vi "Load Layout By Name.vi"(8 "error in (no error)":errorcluster, 10 "key":string, 11 "Cluster":T6) -> (0 "error out":errorcluster)   [LabVIEW 2020, in "MDI ViewManager.lvlib"]
uses:
  MDI ViewManager.lvlib
  Typedef/Layout.ctl
  <vilib>/Utility/miscctls.llb/LVPointTypeDef.ctl
  <vilib>/Utility/miscctls.llb/LVBoundsTypeDef.ctl
  <vilib>/Utility/miscctls.llb/LVPositionTypeDef.ctl
  Typedef/Update View.ctl
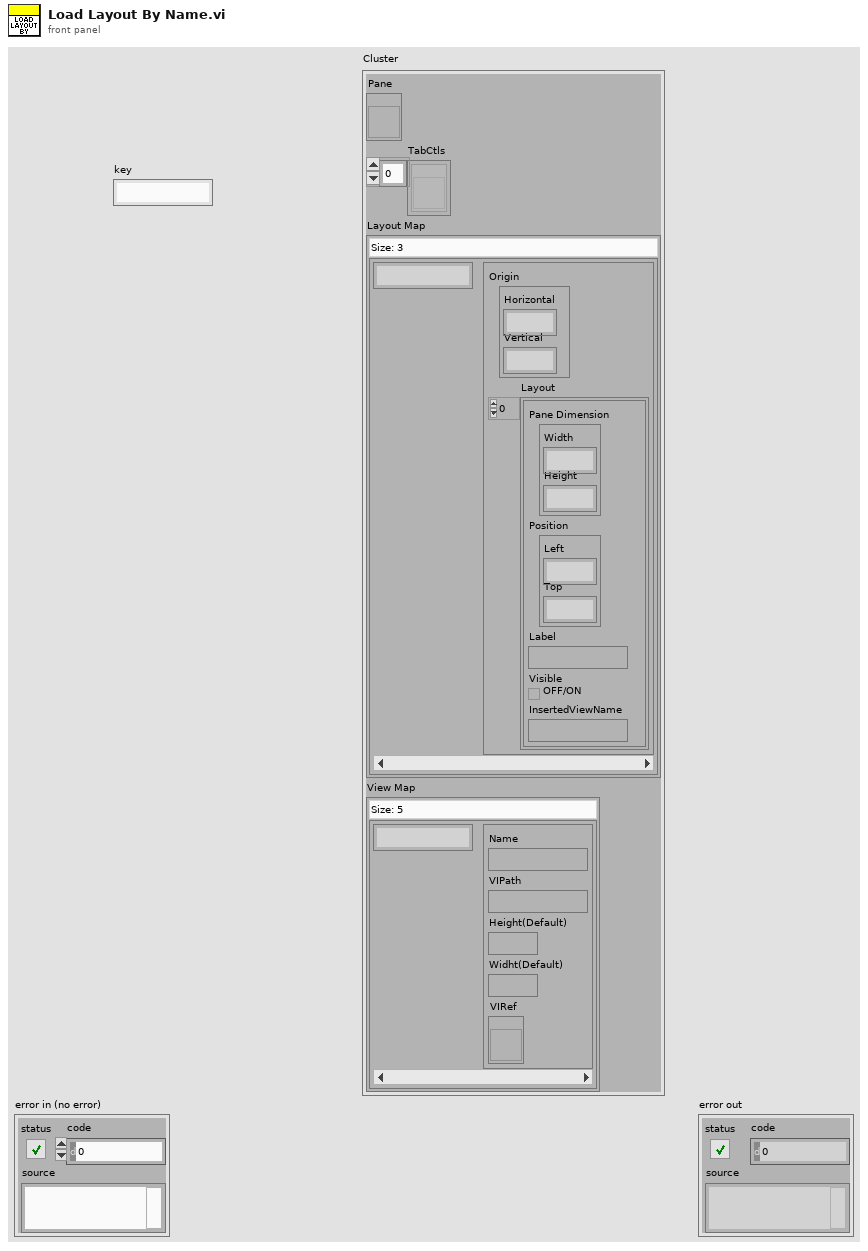
[diagram p1: front panel]
types:
  T1 = typedef "MDI ViewManager.lvlib/Layout.ctl" = cluster{"Origin":T2, "Layout":cluster{"Pane Dimension":T3, "Position":T4, "Label":string, "Visible":bool, "InsertedViewName":string}[]}
  T2 = typedef "LVPointTypeDef.ctl" = cluster{"Horizontal":i16, "Vertical":i16}
  T3 = typedef "LVBoundsTypeDef.ctl" = cluster{"Width":u32, "Height":u32}
  T4 = typedef "LVPositionTypeDef.ctl" = cluster{"Left":i32, "Top":i32}
  T5 = typedef "MDI ViewManager.lvlib/Update View.ctl" = cluster{"Name":string, "VIPath":path, "Height(Default)":u32, "Widht(Default)":u32, "VIRef":refnum<vi>}
  T6 = cluster{"Pane":refnum<vi>, "TabCtls":refnum<vi>[], "Layout Map":map{string, T1}, "View Map":map{string, T5}}
  T7 = cluster{"Pane Dimension":T3, "Position":T4, "Label":string, "Visible":bool, "InsertedViewName":string}[]
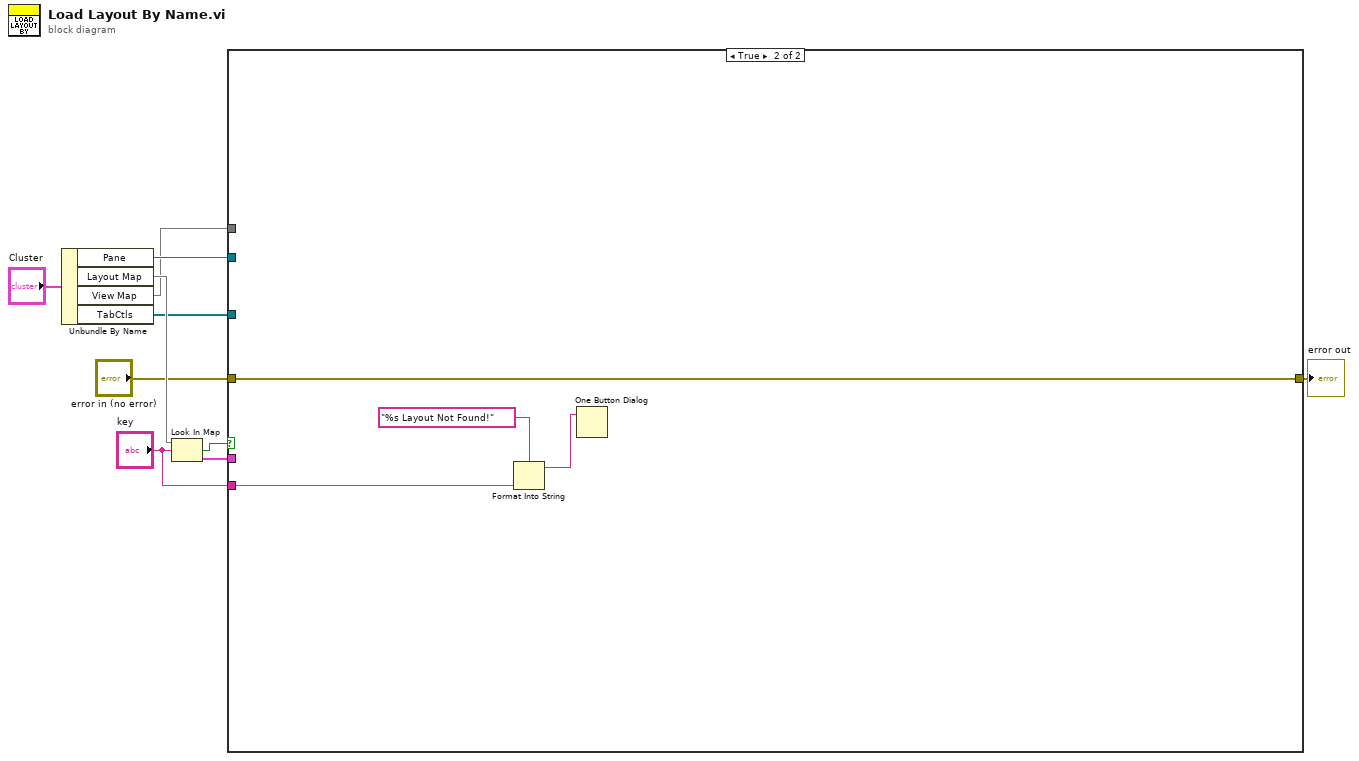
[diagram p0: block diagram]
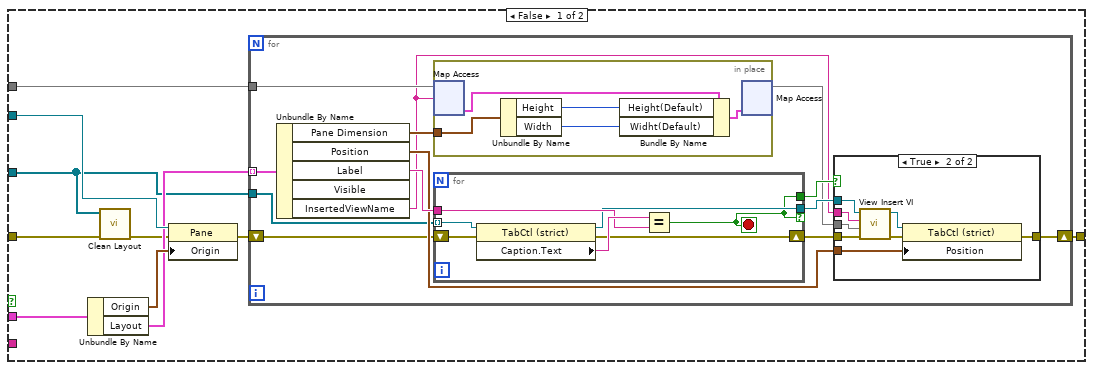
[diagram p2: hidden frame]
diagram:
  n1 = Unbundle By Name("Cluster") -> ("Pane"=w9:refnum<vi>, "Layout Map"=w8:map{string, T1}, "View Map"=w6:map{string, T5}, "TabCtls"=w3:refnum<vi>[])
  n2 = Look In Map(map=w8, key="key") -> (key not found?=w2:bool, value=w7:T1)  [unwired: 1 in]
  n3 = case shown="True" w2 {
    tunnel: w9 -> [w20 _]
    tunnel: w7 -> [w19 _]
    tunnel: w6 -> [w16 _]
    tunnel: [w14 w58] -> w5
    tunnel: "error in (no error)" -> [w13 w58]
    tunnel: w3 -> [w11 _]
    tunnel: "key" -> [_ w56]
    frame False {
      n4 = Unbundle By Name(w19) -> ("Origin"=w18:T2, "Layout"=w17:T7)
      n5 = call "Clean Layout.vi"("error in (no error)"=w13, "TabCtls"=w11) -> ("error out"=w12:errorcluster)  [unwired: 9 in]
      n6 = property class="Pane"(reference=w20, error in=w12, "Origin"=w18) -> (error out=w15:errorcluster)  [unwired: 1 out]
      n7 = for {
        tunnel: w17 -> [w33] mode=indexing
        tunnel: w11 -> [w21]
        tunnel: w16 -> [w30]
        shift-right: [w26] -> w14
        shift-left: w15 -> [w24]
        n8 = Unbundle By Name(w33) -> ("Pane Dimension"=w28:T3, "Position"=w25:T4, "Label"=w29:string, "InsertedViewName"=w22:string)  [unwired: 1 out]
        n9 = in-place {
          in-place-border: w28 -> [w36]
          n10 = in-place-map #1(w30, w22) -> (w38:T5)  [unwired: 1 in, 1 out]
          n11 = Unbundle By Name(w36) -> ("Height"=w35:u32, "Width"=w34:u32)
          n12 = Bundle By Name(cluster=w38, "Height(Default)"=w35, "Widht(Default)"=w34) -> (w37:T5)
          n13 = in-place-map #1(w37) -> (w27:map{string, T5})  [unwired: 1 in, 2 out]
        }
        n14 = for {
          tunnel: w21 -> [w54] mode=indexing
          tunnel: w29 -> [w52]
          tunnel: [w51] -> w31 if=w48
          tunnel: [w48] -> w32
          shift-right: [w50] -> w23
          shift-left: w24 -> [w49]
          stop <- w48 stop-if-true
          n15 = property class="TabCtl (strict)"(reference=w54, error in=w49) -> (reference out=w51:refnum<vi>, error out=w50:errorcluster, "Caption.Text"=w53:string)
          n16 = Equal?(x=w53, y=w52) -> (x = y?=w48:bool)
        }
        n17 = case shown="True" w32 {
          tunnel: w22 -> [_ w40]
          tunnel: w27 -> [_ w47]
          tunnel: w31 -> [_ w46]
          tunnel: [w39 w42] -> w26
          tunnel: w25 -> [_ w45]
          tunnel: w23 -> [w39 w41]
          frame False {
          }
          frame True {
            n18 = call "View Insert VI.vi"("error in (no error)"=w41, "ViewMap"=w47, "Name"=w40, "TabControl in"=w46) -> ("error out"=w43:errorcluster, "TabControl in 2"=w44:refnum<vi>)  [unwired: 6 in]
            n19 = property class="TabCtl (strict)"(reference=w44, error in=w43, "Position"=w45) -> (error out=w42:errorcluster)  [unwired: 1 out]
          }
        }
      }
    }
    frame True {
      n20 = Format Into String(format string="%s Layout Not Found!" ("message"), w56) -> (resulting string=w55:string)  [unwired: 2 in, 1 out]
      n21 = One Button Dialog(message=w55) -> ()  [unwired: 1 in, 1 out]
    }
  }
  "error out" <- w5
